vi "get_points.vi"(7 "retrieval mode":T1, 8 "error in (no error)":errorcluster, 11 "PointCollection in":refnum<class "PointCollection.lvclass">) -> (0 "error out":errorcluster, 2 "points":dbl[][](array[numeric]), 3 "PointCollection out":refnum<class "PointCollection.lvclass">)   [LabVIEW 2010, in "PointCollection.lvclass"]
uses:
  PointCollection.lvclass
  mode_enum.ctl
  PointCollection.lvclass/PointCollection.ctl
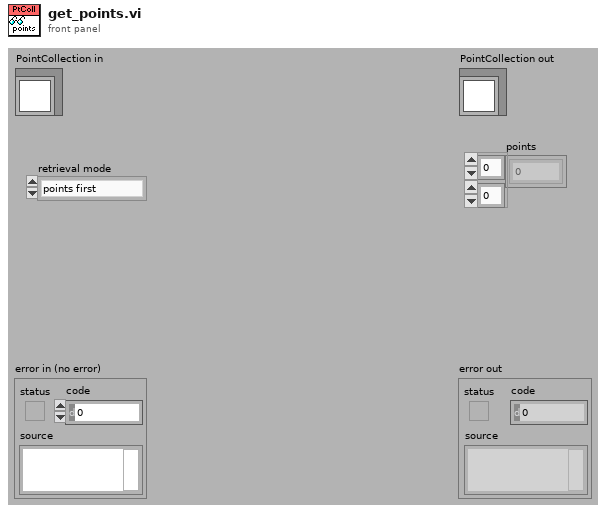
[diagram p1: front panel]
types:
  T1 = typedef "PointCollection.lvclass/mode_enum.ctl" = enum16{"points first", "dimensions first"}
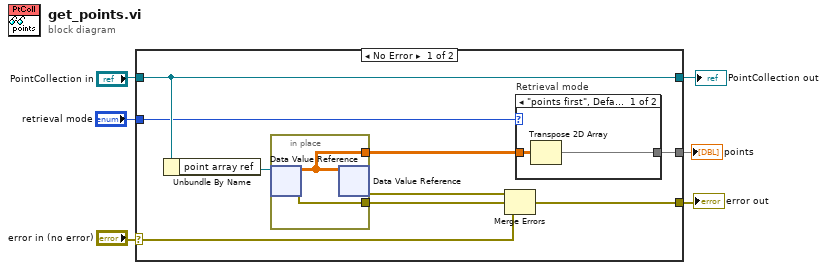
[diagram p0: block diagram]
diagram:
  n1 = case shown="No Error" "error in (no error)" {
    selector: "error in (no error)" -> [w10 w22]
    tunnel: [w11 w22] -> w5
    tunnel: [w15 w21] -> w6
    tunnel: "PointCollection in" -> [w15 w21]
    tunnel: [w9 _] -> w2
    tunnel: "retrieval mode" -> [w7 _]
    frame No Error {
      n2 = Unbundle By Name(w15) -> ("point array ref"=w14:refnum<data-value>)
      n3 = in-place {
        in-place-border: [w20] -> w8
        in-place-border: [w19] -> w13
        n4 = in-place-dvr #1(w14) -> (w20:dbl[][], w19:errorcluster)
        n5 = in-place-dvr #1(w20) -> (w12:errorcluster)  [unwired: 1 out]
      }
      n6 = Merge Errors(w12, w13, w10) -> (w11:errorcluster)
      n7 = case "Retrieval mode" shown="\"points first\", Default" w7 {
        tunnel: [w17 w18] -> w9
        tunnel: w8 -> [w16 w18]
        frame "points first", Default {
          n8 = Transpose 2D Array(2D array=w16) -> (transposed array=w17:dbl[][])
        }
        frame "dimensions first" {
        }
      }
    }
    frame Error {
    }
  }
  "error out" <- w5
  "PointCollection out" <- w6
  "points" <- w2
